vi "题目2.vi"() -> ()   [LabVIEW 2017]
panel:
  out "注册":bool
  in  "簇":cluster{"注册":bool, "姓名":string, "学号":dbl}
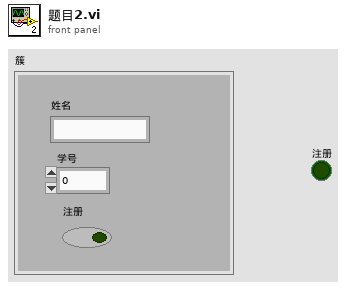
[diagram p1: front panel]
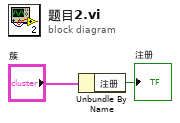
[diagram p0: block diagram]
diagram:
  n1 = Unbundle By Name("簇") -> ("注册"=→"注册":bool)
